vi "Excel Macro Example.vi"() -> ()   [LabVIEW 2014]
doc: "注：运行该范例需要Excel 97或更高版本。\n\n本VI将创建一个二维数组并传地至Excel，然后运行名为GraphData的Excel宏。数组的第一列和第二列分别为时间和日期。GraphData宏已被预定义。如需查看该宏的代码，请选择工具>>宏>>宏，在结果对话框中选择GraphData并单击编辑按钮。\n\n运行本范例前，请确保project.xls位于本VI的相同目录中。"
panel:
  in  "Workbook Name":string="project.xls" caption="工作簿名称"
  in  "dt":dbl=0.25 format="%0.2f"
  in  "Data Values":dbl[](array[numeric])=[0.0, 1.0, 2.0, 3.0, 4.0, 5.0] caption="数据值" format="%0.2f"
  # "请确保该文件与范例VI处于\n相同目录中。"
  # "注:\n运行该范例需要Excel 97或\n更高版本。"
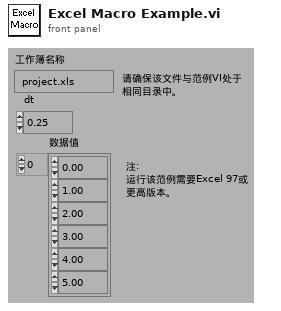
[diagram p1: front panel]
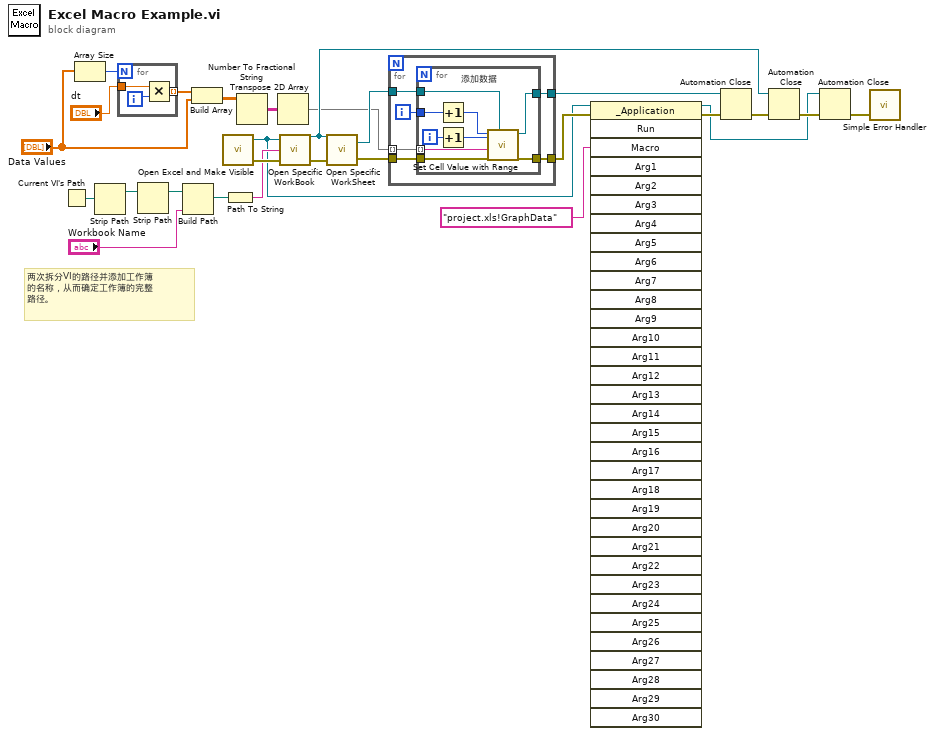
[diagram p0: block diagram]
diagram:
  # "两次拆分VI的路径并添加工作簿\n的名称，从而确定工作簿的完整\n路径。"
  n1 = Current VI's Path() -> (path=w8:path)
  n2 = Array Size(array="Data Values") -> (size(s)=w19:i32)
  n3 = Strip Path(path=w8) -> (stripped path=w7:path)  [unwired: 1 out]
  n4 = for {
    N: w19 -> [_]
    tunnel: "dt" -> [w30]
    tunnel: [w28] -> w23 mode=indexing
    i -> [w29]
    n5 = Multiply(x=w30, y=w29) -> (x*y=w28:dbl)
  }
  n6 = Strip Path(path=w7) -> (stripped path=w6:path)  [unwired: 1 out]
  n7 = Build Path(base path=w6, name or relative path="Workbook Name") -> (appended path=w4:path)
  n8 = Build Array(w23, "Data Values") -> (w22:dbl[][])
  n9 = call "Open Excel and Make Visible.vi"() -> ("error out"=w26:errorcluster, "Excel._Application"=w1:refnum<k7>)  [unwired: 2 in]
  n10 = Path To String(path=w4) -> (string=w9:string)
  n11 = Number To Fractional String(number=w22) -> (F-format string=w21:string[][])  [unwired: 3 in]
  n12 = Transpose 2D Array(2D array=w21) -> (transposed array=w2:string[][])
  n13 = call "Open Specific WorkBook.vi"("error in (no error)"=w26, "Filename of Workbook"=w9, "Excel._Application"=w1) -> ("error out"=w27:errorcluster, "Excel._Workbook"=w16:refnum<k7>)
  n14 = call "Open Specific WorkSheet.vi"("error in (no error)"=w27, "Excel._Workbook"=w16) -> ("error out"=w25:errorcluster, "Excel._Worksheet"=w18:refnum<k7>)  [unwired: 1 in]
  n15 = for {
    tunnel: w18 -> [w36]
    tunnel: w25 -> [w34]
    tunnel: w2 -> [w33] mode=indexing
    tunnel: [w32] -> w17
    tunnel: [w31] -> w10
    i -> [w35]
    n16 = for {
      tunnel: w36 -> [w44]
      tunnel: w34 -> [w43]
      tunnel: [w42] -> w31
      tunnel: w35 -> [w41]
      tunnel: w33 -> [w40] mode=indexing
      tunnel: [w39] -> w32
      i -> [w45]
      # "添加数据"
      n17 = Increment(x=w41) -> (x+1=w38:i32)
      n18 = Increment(x=w45) -> (x+1=w37:i32)
      n19 = call "Set Cell Value with Range.vi"("Excel._Worksheet"=w44, "error in (no error)"=w43, "Value"=w40, "Col"=w37, "Row"=w38) -> ("error out"=w42:errorcluster, "Excel._Worksheet"=w39:refnum<k7>)  [unwired: 2 out]
    }
  }
  n20 = invoke class="_Application" method="Run"(reference=w1, error in=w10, "Macro"="project.xls!GraphData") -> (reference out=w3:refnum<k7>, error out=w11:errorcluster)  [unwired: 31 in, 32 out]
  n21 = Automation Close(3:w11, 5:w17) -> (0:w15:errorcluster)
  n22 = Automation Close(3:w15, 5:w16) -> (0:w14:errorcluster)
  n23 = Automation Close(3:w14, 5:w3) -> (0:w13:errorcluster)
  n24 = call <vilib>:"Simple Error Handler.vi"("error in (no error)"=w13) -> ()  [unwired: 4 in, 5 out]
